vi "Plot menu activation_.vi"(7 "menu tag":string, 8 "error in (no error)":errorcluster, 10 "MenuRef":refnum<k9>, 11 "StokePlotHandle in":refnum<class "BjusticePlotHandle.lvclass">) -> (0 "error out":errorcluster, 2 "MenuRef":refnum<k9>, 3 "StokePlotHandle out":refnum<class "BjusticePlotHandle.lvclass">)   [LabVIEW 2021, in "BjusticePlotHandle.lvclass"]
uses:
  BjusticePlotHandle.lvclass
  BjusticePlotHandle.lvclass/BjusticePlotHandle.ctl
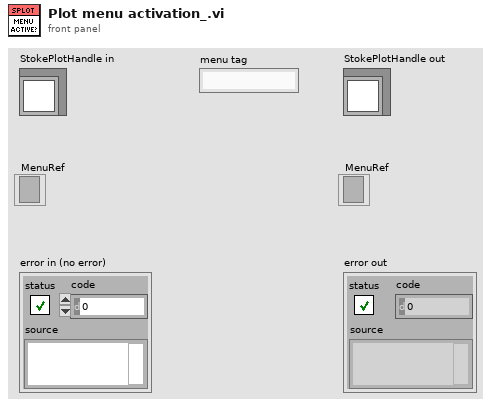
[diagram p1: front panel]
types:
  T1 = typedef "StokePlotHandle.lvclass/Type.ctl" = enum16{"1PLOT", "MPLOT"}
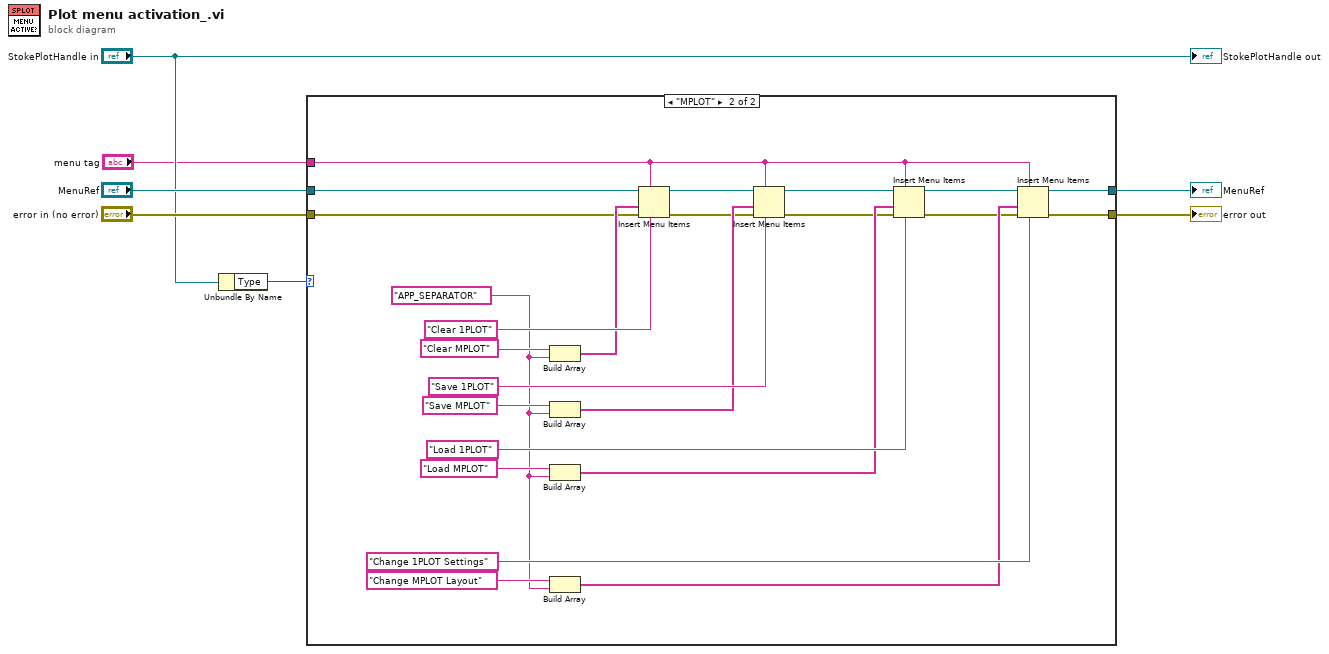
[diagram p0: block diagram]
diagram:
  n1 = Unbundle By Name("StokePlotHandle in") -> ("Type"=w2:T1)
  n2 = case shown="\"MPLOT\"" w2 {
    tunnel: "MenuRef" -> [w9 w33]
    tunnel: [w9 w17] -> w6
    tunnel: "error in (no error)" -> [w8 w16]
    tunnel: [w8 w13] -> w4
    tunnel: "menu tag" -> [_ w12]
    frame "1PLOT" {
    }
    frame "MPLOT" {
      w23 = "APP_SEPARATOR"
      n3 = Build Array("Clear MPLOT", w23) -> (w27:string[])
      n4 = Build Array("Save MPLOT", w23) -> (w22:string[])
      n5 = Build Array("Load MPLOT", w23) -> (w21:string[])
      n6 = Build Array("Change MPLOT Layout", w23) -> (w20:string[])
      n7 = Insert Menu Items(4:"Clear 1PLOT", 5:w12, 6:w16, 7:w27, 9:w33) -> (0:w15:errorcluster, 3:w19:refnum<k9>)  [unwired: 1 in, 1 out]
      n8 = Insert Menu Items(4:"Save 1PLOT", 5:w12, 6:w15, 7:w22, 9:w19) -> (0:w14:errorcluster, 3:w18:refnum<k9>)  [unwired: 1 in, 1 out]
      n9 = Insert Menu Items(4:"Load 1PLOT", 5:w12, 6:w14, 7:w21, 9:w18) -> (0:w11:errorcluster, 3:w10:refnum<k9>)  [unwired: 1 in, 1 out]
      n10 = Insert Menu Items(4:"Change 1PLOT Settings", 5:w12, 6:w11, 7:w20, 9:w10) -> (0:w13:errorcluster, 3:w17:refnum<k9>)  [unwired: 1 in, 1 out]
    }
  }
  "error out" <- w4
  "MenuRef" <- w6
  "StokePlotHandle out" <- "StokePlotHandle in"
